vi "TreeController.vi"(8 "SaveHistory":bool, 10 "Tree Refnum":refnum<vi>, 11 "Commands":refnum<queue>) -> ()   [LabVIEW 2021, in "Tree.lvlib" / "Tree.lvclass"]
uses:
  Tree.lvclass
  TreeController.ctl
  TreeData.ctl
  <vilib>/Utility/miscctls.llb/LVNodeAndColumnTypeDef.ctl
  Tree.lvclass/Tree.ctl
panel:
  in  "exit":bool
  in  "Cluster":T1
  out "Mode":enum8{"AND", "OR", "NOT AND", "NOT OR"}(ring)
  out "Filter":cluster{"Matches String":string, "Column":i32}[](array[cluster])
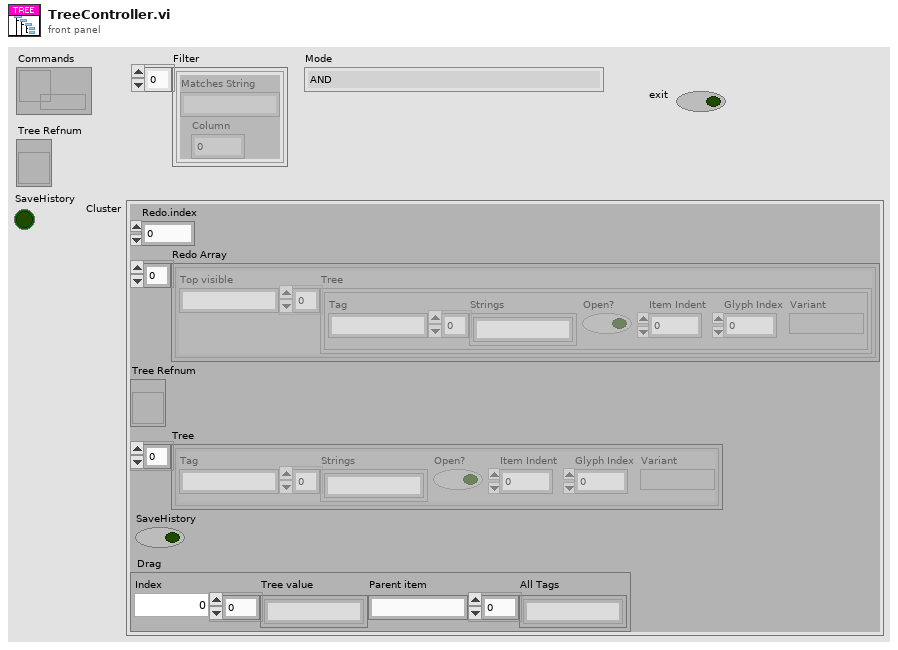
[diagram p1: front panel]
types:
  T1 = typedef "Tree.lvlib/Tree.lvclass/TreeController.ctl" = cluster{"Redo.index":i32, "Redo Array":cluster{"Top visible":string, "Tree":T2[]}[], "Tree Refnum":refnum<vi>, "Tree":T2[], "SaveHistory":bool, "Drag":cluster{"Index":i32, "Tree value":string[], "Parent item":string, "All Tags":string[]}}
  T2 = typedef "Tree.lvlib/Tree.lvclass/TreeData.ctl" = cluster{"Tag":string, "Strings":string[], "Open?":bool, "Item Indent":i32, "Glyph Index":i32, "Variant":variant}
  T3 = cluster{"NewElement":cluster{"SelectedTag":string, "New Tag":string, "Strings":string[], "Child?":bool, "Variant":variant}, "queue out":refnum<queue>}
  T4 = cluster{"Tag":string[], "queue out":refnum<queue>}
  T5 = cluster{"Tag":string, "Strings":string[], "Open?":bool, "Item Indent":i32, "Glyph Index":i32, "Variant":variant}
  T6 = cluster{"Tree":T2[], "Mode":enum16{"Clear & Insert", "Update Existing", "Add to End"}}
  T7 = cluster{"Tags":string[], "queue out":refnum<queue>}
  T8 = cluster{"cluster":cluster{enum16{"EditStrings", "EditGraph", "EditVariant"}, "Tag":string, "Value":variant}, "queue out":refnum<queue>}
  T9 = cluster{"T=Back F=Forward":bool, "queue out":refnum<queue>}
  T10 = typedef "LVNodeAndColumnTypeDef.ctl" = cluster{"Node":string, "Column":i32}
  T11 = enum8{"Enabled", "Disabled", "Disabled and Grayed Out"}
  T12 = cluster{"Mode":enum8{"AND", "OR", "NOT AND", "NOT OR"}, "Filter":cluster{"Matches String":string, "Column":i32}[], "Show Hierarhy":cluster{"Show hierarhy in first column(F)":bool, "Left separator":string, "Right separator":string}}
  T13 = cluster{"SelectedTag":string, "New Tag":string, "Strings":string[], "Child?":bool, "Variant":variant}
  T14 = cluster{"StepBack":enum8{"Enabled", "Disabled", "Disabled and Grayed Out"}, "StepForward":enum8{"Enabled", "Disabled", "Disabled and Grayed Out"}, "Edit Tree Items:Add Item":string}
  T15 = cluster{"StepBack":enum8{"Enabled", "Disabled", "Disabled and Grayed Out"}, "StepForward":enum8{"Enabled", "Disabled", "Disabled and Grayed Out"}}
  T16 = cluster{"Node":string, cluster{"Tag":string, "Strings":string[], "Open?":bool, "Item Indent":i32, "Glyph Index":i32, "Variant":variant}[]}
  T17 = enum16{"Clear & Insert", "Update Existing", "Add to End"}
  T18 = cluster{enum16{"EditStrings", "EditGraph", "EditVariant"}, "Tag":string, "Value":variant}
  T19 = enum16{"EditStrings", "EditGraph", "EditVariant"}
  T20 = cluster{"Disabled & Grayed":enum8{"Enabled", "Disabled", "Disabled and Grayed Out"}, "Disabled & Grayed":enum8{"Enabled", "Disabled", "Disabled and Grayed Out"}}
  T21 = cluster{"Show hierarhy in first column(F)":bool, "Left separator":string, "Right separator":string}
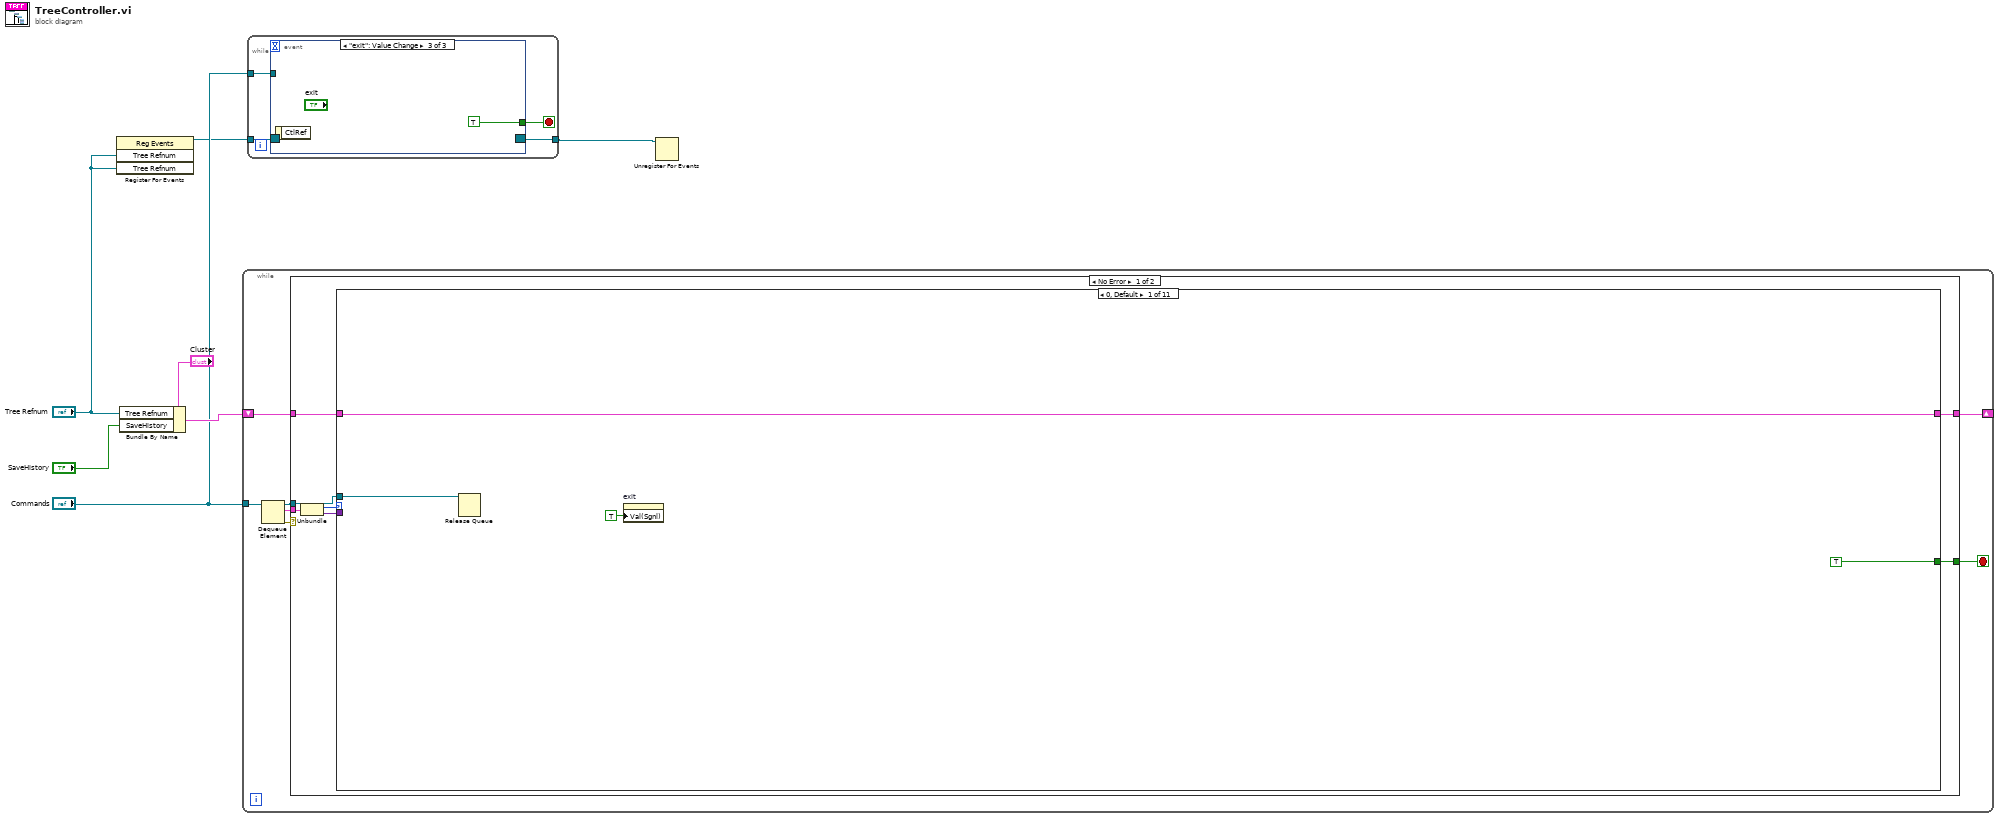
[diagram p0: block diagram]
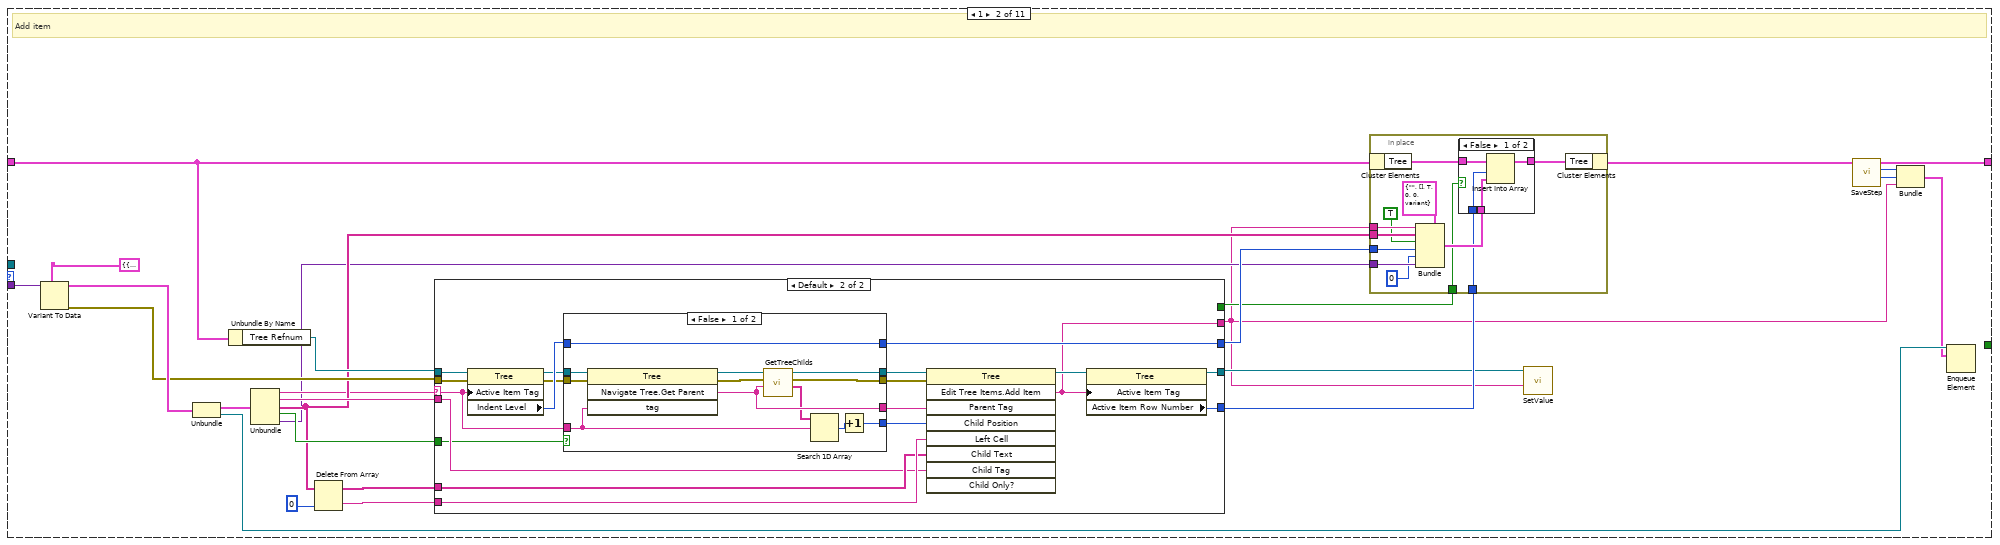
[diagram p2: hidden frame]
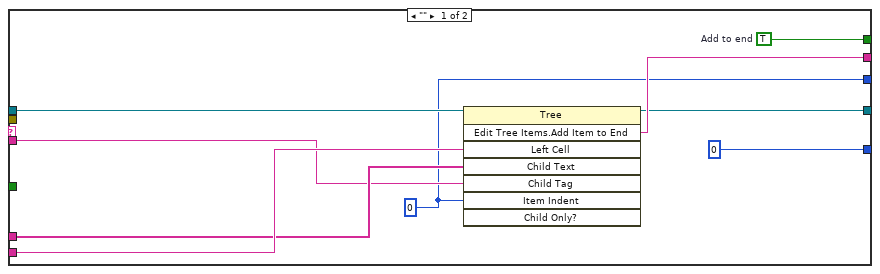
[diagram p3: hidden frame]
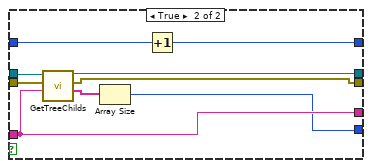
[diagram p4: hidden frame]
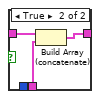
[diagram p5: hidden frame]
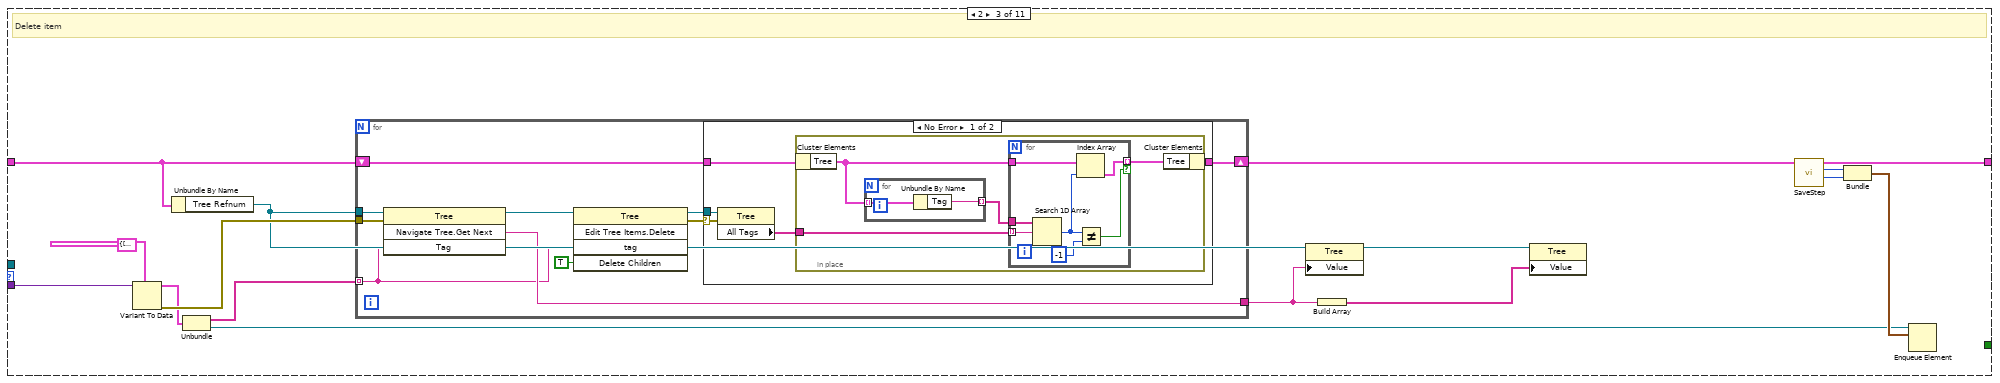
[diagram p6: hidden frame]
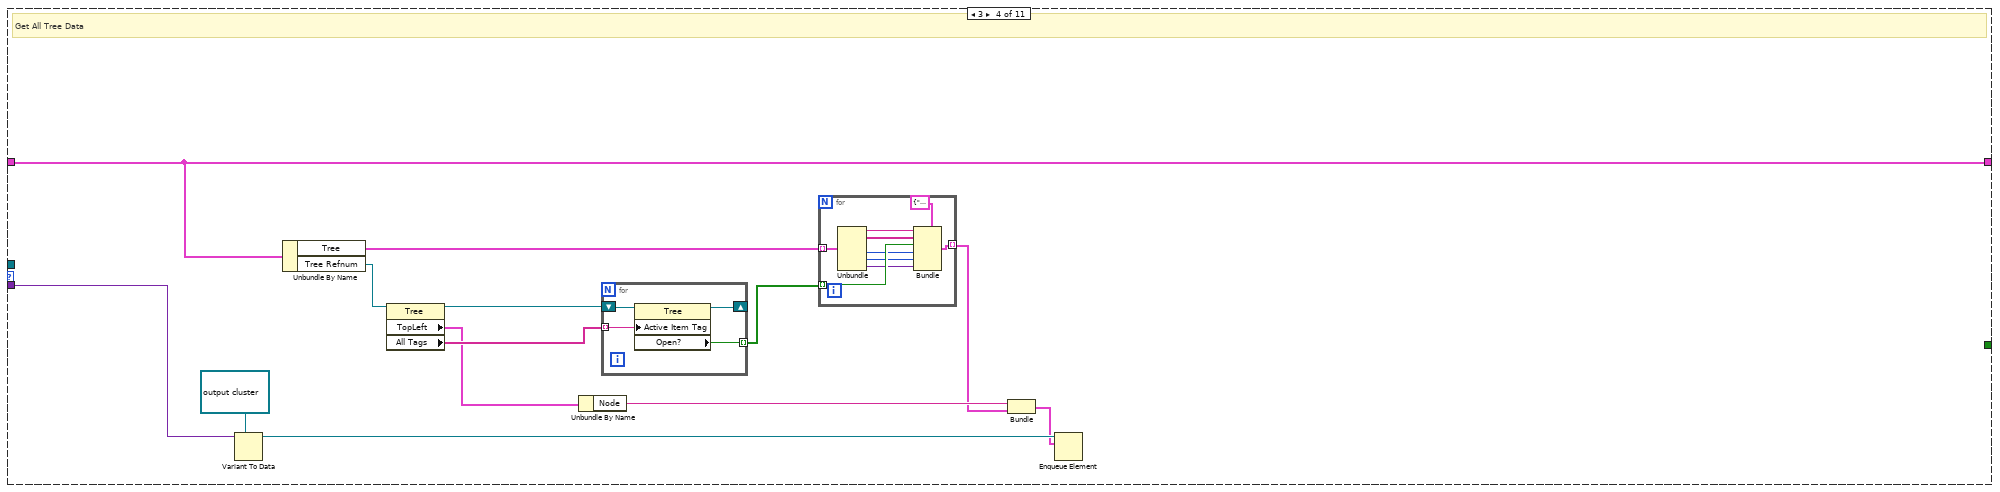
[diagram p8: hidden frame]
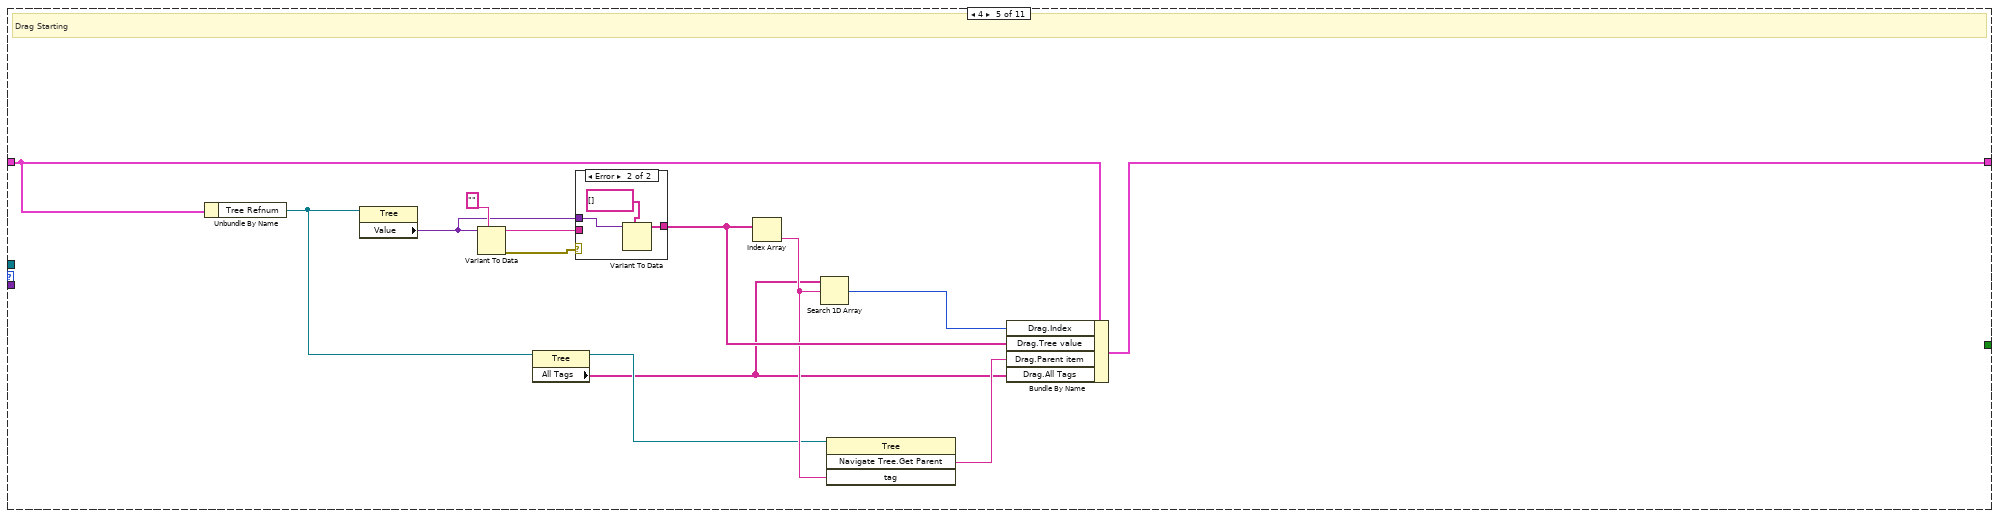
[diagram p9: hidden frame]
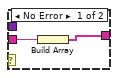
[diagram p10: hidden frame]
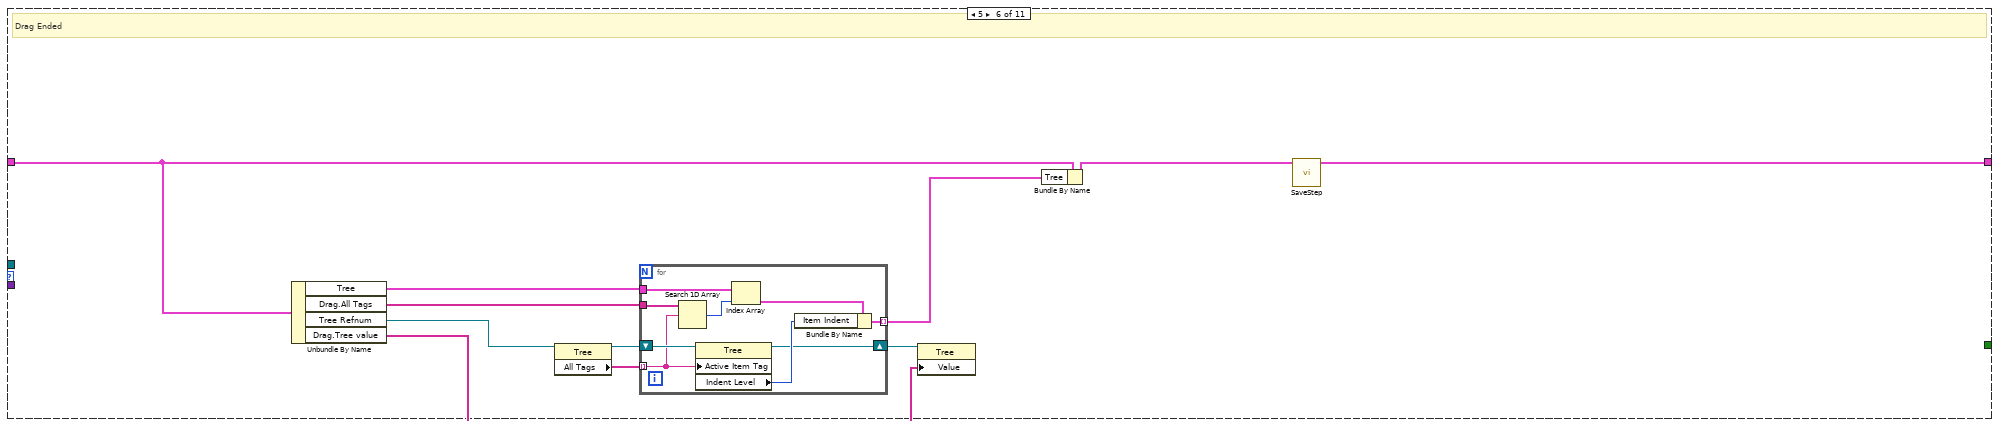
[diagram p11: hidden frame]
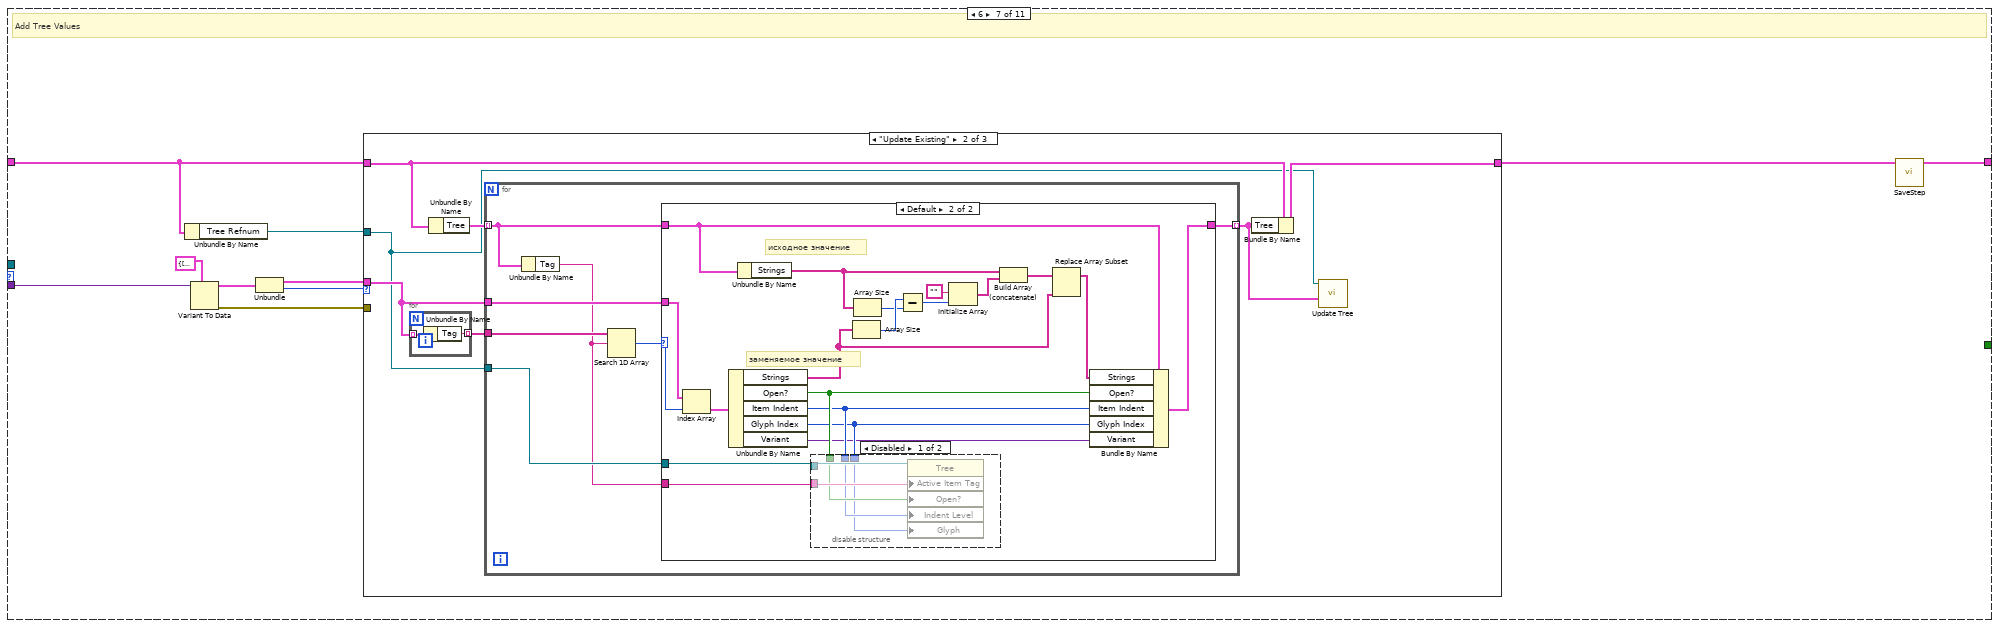
[diagram p12: hidden frame]
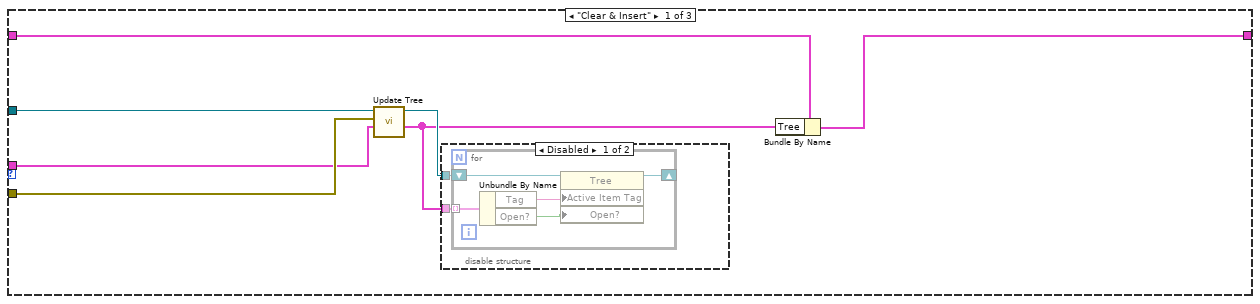
[diagram p13: hidden frame]
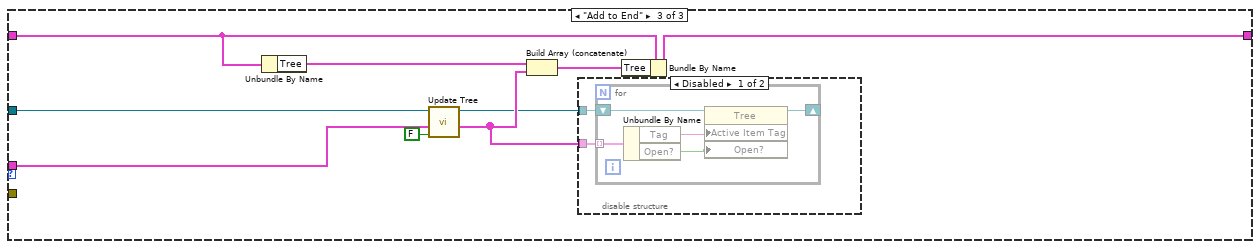
[diagram p17: hidden frame]
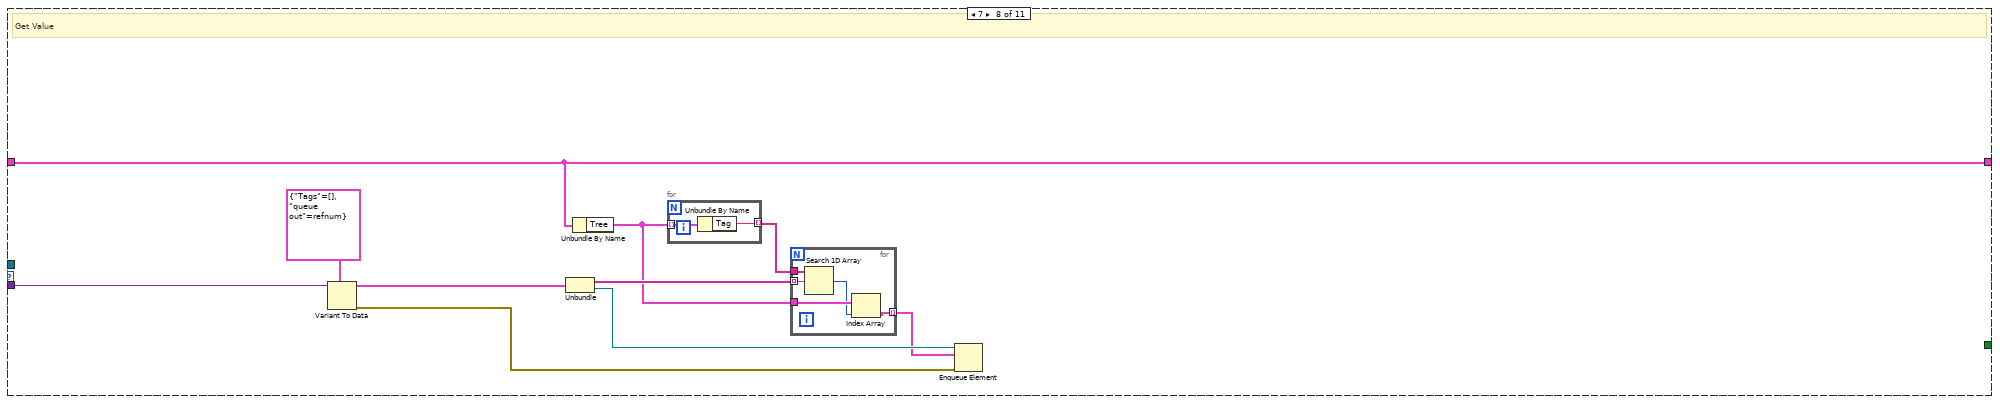
[diagram p19: hidden frame]
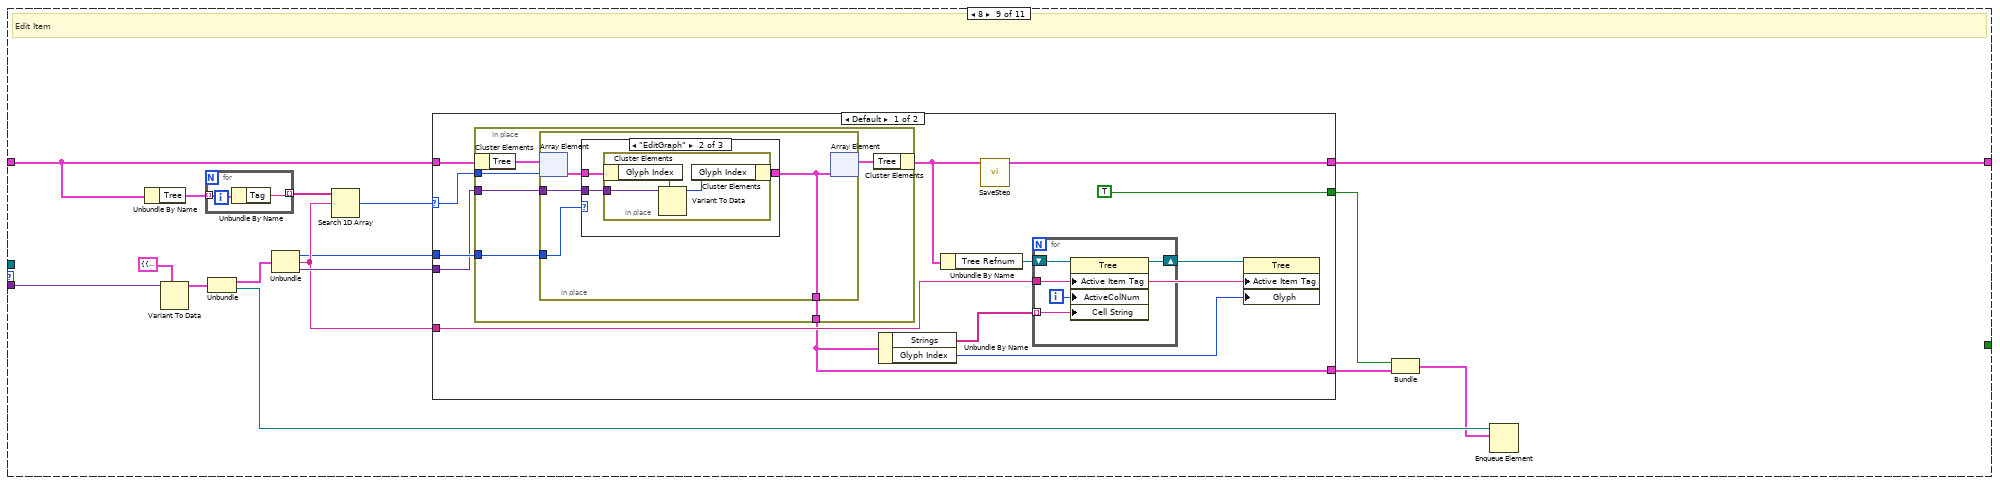
[diagram p20: hidden frame]
diagram:
  n1 = register-events("Tree Refnum", "Tree Refnum") -> (reference out=w2:refnum<event-registration>)  [unwired: 2 in, 1 out]
  n2 = Bundle By Name(cluster="Cluster", "Tree Refnum"="Tree Refnum", "SaveHistory"="SaveHistory") -> (w6:T1)
  n3 = while {
    tunnel: "Commands" -> [w14]
    shift-right: [w12] -> _
    shift-left: w6 -> [w11]
    stop <- w9 stop-if-true
    n4 = Dequeue Element(queue=w14) -> (queue out=w8:refnum<queue>, element=w13:cluster{"Tag":u8, "Value":variant}, error out=w10:errorcluster)  [unwired: 2 in, 1 out]
    n5 = case shown="No Error" w10 {
      selector: w10 -> [_ w508]
      tunnel: w13 -> [w21 _]
      tunnel: [w19 w510] -> w12
      tunnel: w11 -> [w18 w510]
      tunnel: [w16 TRUE] -> w9
      tunnel: w8 -> [w15 _]
      frame No Error {
        n6 = Unbundle(w21) -> ("Tag"=w20:u8, "Value"=w17:variant)
        n7 = case shown="0, Default" w20 {
          tunnel: [w23 w50 w132 w177 w198 w219 w235 w318 w337 w410 w449] -> w19
          tunnel: w18 -> [w23 w51 w134 w177 w203 w218 w238 w318 w338 w423 w449]
          tunnel: w17 -> [_ w49 w135 w173 _ _ w234 w320 w343 w424 w445]
          tunnel: [TRUE _ _ _ _ _ _ _ _ _ _] -> w16
          tunnel: w15 -> [w24 _ _ _ _ _ _ _ _ _ _]
          frame 0, Default {
            n8 = Release Queue(queue=w24) -> ()  [unwired: 2 in, 3 out]
            n9 = property on="exit" class="Bool (strict)"("Val(Sgnl)"=TRUE ("Value (Signaling)")) -> ()  [unwired: 2 in, 2 out]
          }
          frame 1 {
            # "Add item"
            n10 = Variant To Data(type=T3 {"NewElement"={"SelectedTag"="", "New Tag"="", "Strings"=[], "Child?"=FALSE, "Variant"=variant}, "queue out"=refnum} ("output cluster"), Variant=w49) -> (data=w48:T3, error out=w46:errorcluster)  [unwired: 1 in]
            n11 = Unbundle(w48) -> ("NewElement"=w35:T13, "queue out"=w36:refnum<queue>)
            n12 = Unbundle By Name(w51) -> ("Tree Refnum"=w38:refnum<vi>)
            n13 = Unbundle(w35) -> ("SelectedTag"=w29:string, "New Tag"=w42:string, "Strings"=w30:string[], "Child?"=w39:bool, "Variant"=w28:variant)
            n14 = Delete From Array(array=w30, index=0) -> (deleted portion=w45:string, array with subset deleted=w44:string[])  [unwired: 1 in]
            n15 = case shown="Default" w29 {
              selector: w29 -> [_ w62]
              tunnel: w45 -> [w59 w79]
              tunnel: w44 -> [w58 w78]
              tunnel: [w53 w77] -> w43
              tunnel: w42 -> [w54 w76]
              tunnel: [0 ("Active Item Row Number") w75] -> w41
              tunnel: w39 -> [_ w69]
              tunnel: w38 -> [w56 w68]
              tunnel: w46 -> [_ w64]
              tunnel: [w57 w63] -> w26
              tunnel: [w55 _] -> w34
              tunnel: [w52 w61] -> w27
              frame "" {
                w55 = TRUE  # Add to end
                w53 = 0 ("New Item Indentation")
                n16 = invoke class="Tree" method="Edit Tree Items.Add Item to End"(reference=w56, "Left Cell"=w59, "Child Text"=w58, "Child Tag"=w54, "Item Indent"=w53) -> (reference out=w52:refnum<vi>, "Edit Tree Items:Add Item to End"=w57:string)  [unwired: 3 in, 6 out]
              }
              frame Default {
                n17 = property class="Tree"(reference=w68, error in=w64, "Active Item Tag"=w62) -> (reference out=w66:refnum<vi>, error out=w65:errorcluster, "Indent Level"=w67:i32)
                n18 = case shown="False" w69 {
                  tunnel: [w80 w92] -> w77
                  tunnel: w65 -> [w89 w94]
                  tunnel: w62 -> [w91 w99]
                  tunnel: w66 -> [w90 w100]
                  tunnel: [w87 w99] -> w74
                  tunnel: [w85 w95] -> w73
                  tunnel: [w84 w96] -> w72
                  tunnel: [w81 w97] -> w71
                  tunnel: w67 -> [w80 w93]
                  frame False {
                    n19 = invoke class="Tree" method="Navigate Tree.Get Parent"(reference=w90, error in=w89, "tag"=w91) -> (reference out=w88:refnum<vi>, error out=w86:errorcluster, "Navigate Tree:Get Parent"=w87:string)  [unwired: 1 in, 1 out]
                    n20 = call "GetTreeChilds.vi"("Tag"=w87, "error in (no error)"=w86, "Tree Refnum"=w88) -> ("Childs"=w83:string[], "error out"=w85:errorcluster, "Tree Refnum"=w84:refnum<vi>)  [unwired: 6 in]
                    n21 = Search 1D Array(1D array=w83, element=w91) -> (index of element=w82:i32)  [unwired: 1 in]
                    n22 = Increment(x=w82) -> (x+1=w81:i32)
                  }
                  frame True {
                    n23 = call "GetTreeChilds.vi"("Tag"=w99, "error in (no error)"=w94, "Tree Refnum"=w100) -> ("Childs"=w98:string[], "error out"=w95:errorcluster, "Tree Refnum"=w96:refnum<vi>)  [unwired: 6 in]
                    n24 = Array Size(array=w98) -> (size(s)=w97:i32)
                    n25 = Increment(x=w93) -> (x+1=w92:i32)
                  }
                }
                n26 = invoke class="Tree" method="Edit Tree Items.Add Item"(reference=w72, error in=w73, "Parent Tag"=w74, "Child Position"=w71, "Left Cell"=w79, "Child Text"=w78, "Child Tag"=w76) -> (reference out=w70:refnum<vi>, "Edit Tree Items:Add Item"=w63:string)  [unwired: 2 in, 7 out]
                n27 = property class="Tree"(reference=w70, "Active Item Tag"=w63) -> (reference out=w61:refnum<vi>, "Active Item Row Number"=w75:i32)  [unwired: 1 in, 1 out]
              }
            }
            n28 = in-place {
              in-place-border: w26 -> [w111]
              in-place-border: w30 -> [w110]
              in-place-border: w43 -> [w109]
              in-place-border: w41 -> [w106]
              in-place-border: w34 -> [w105]
              in-place-border: w28 -> [w104]
              n29 = in-place-cluster #1(w51) -> ("Tree"=w112:T2[])
              n30 = Bundle(cluster=T2 {"Tag"="", "Strings"=[], "Open?"=TRUE, "Item Indent"=0, "Glyph Index"=0, "Variant"=variant} ("Item"), "Tag"=w111, "Strings"=w110, "Open?"=TRUE, "Item Indent"=w109, "Glyph Index"=0, "Variant"=w104) -> (w108:T2)
              n31 = case shown="False" w105 {
                tunnel: w112 -> [w116 w119]
                tunnel: w108 -> [w115 w118]
                tunnel: [w114 w117] -> w107
                tunnel: w106 -> [w113 _]
                frame False {
                  n32 = Insert Into Array(array=w116, index=w113, new element=w115) -> (w114:T2[])
                }
                frame True {
                  n33 = Build Array (concatenate)(w119, w118) -> (w117:T2[])
                }
              }
              n34 = in-place-cluster #1("Tree"=w107) -> (w37:T1)
            }
            n35 = call "SetValue.vi"("Edit Tree Items:Add Item"=w26, "TreeControl in"=w27) -> ()  [unwired: 9 in, 1 out]
            n36 = call "SaveStep.vi"("Cluster"=w37) -> ("StepForward"=w32:T11, "StepBack"=w33:T11, "Cluster"=w50:T1)  [unwired: 8 in]
            n37 = Bundle("StepBack"=w33, "StepForward"=w32, "Edit Tree Items:Add Item"=w26) -> (w31:T14)  [unwired: 1 in]
            n38 = Enqueue Element(queue=w36, element=w31) -> ()  [unwired: 2 in, 3 out]
          }
          frame 2 {
            # "Delete item"
            n39 = Variant To Data(type=T4 {"Tag"=[], "queue out"=refnum}, Variant=w135) -> (data=w130:T4, error out=w133:errorcluster)  [unwired: 1 in]
            n40 = Unbundle By Name(w134) -> ("Tree Refnum"=w121:refnum<vi>)
            n41 = Unbundle(w130) -> ("Tag"=w129:string[], "queue out"=w125:refnum<queue>)
            n42 = for {
              tunnel: w121 -> [w140]
              tunnel: w133 -> [w138]
              tunnel: w129 -> [w136] mode=indexing
              shift-right: [w142] -> w124
              shift-left: w134 -> [w144]
              tunnel: [w137] -> w122
              n43 = invoke class="Tree" method="Navigate Tree.Get Next"(reference=w140, error in=w138, "Tag"=w136) -> (reference out=w139:refnum<vi>, "Navigate Tree:Get Next Item"=w137:string)  [unwired: 1 in, 2 out]
              n44 = invoke class="Tree" method="Edit Tree Items.Delete"(reference=w139, "tag"=w136, "Delete Children"=TRUE ("Delete Children?")) -> (reference out=w143:refnum<vi>, error out=w141:errorcluster)  [unwired: 2 in, 3 out]
              n45 = case shown="No Error" w141 {
                selector: w141 -> [w146 _]
                tunnel: w144 -> [w150 w164]
                tunnel: w143 -> [w149 _]
                tunnel: [w147 w164] -> w142
                frame No Error {
                  n46 = property class="Tree"(reference=w149, error in=w146) -> ("All Tags"=w148:string[])  [unwired: 2 out]
                  n47 = in-place {
                    in-place-border: w148 -> [w154]
                    n48 = in-place-cluster #2(w150) -> ("Tree"=w152:T2[])
                    n49 = for {
                      tunnel: w152 -> [w163] mode=indexing
                      tunnel: [w162] -> w153 mode=indexing
                      n50 = Unbundle By Name(w163) -> ("Tag"=w162:string)
                    }
                    n51 = for {
                      tunnel: w154 -> [w160] mode=indexing
                      tunnel: w153 -> [w161]
                      tunnel: w152 -> [w159]
                      tunnel: [w158] -> w151 mode=indexing if=w155
                      n52 = Search 1D Array(1D array=w161, element=w160) -> (index of element=w157:i32)  [unwired: 1 in]
                      n53 = Index Array(array=w159, index=w157) -> (element=w158:T2)
                      n54 = Not Equal?(x=w157, y=-1) -> (x != y?=w155:bool)
                    }
                    n55 = in-place-cluster #2("Tree"=w151) -> (w147:T1)
                  }
                }
                frame Error {
                }
              }
            }
            n56 = property class="Tree"(reference=w121, "Value"=w122) -> (reference out=w120:refnum<vi>)  [unwired: 1 in, 1 out]
            n57 = Build Array(w122) -> (w123:string[])
            n58 = property class="Tree"(reference=w120, "Value"=w123) -> ()  [unwired: 1 in, 2 out]
            n59 = call "SaveStep.vi"("Cluster"=w124) -> ("StepForward"=w126:T11, "StepBack"=w127:T11, "Cluster"=w132:T1)  [unwired: 8 in]
            n60 = Bundle("StepBack"=w127, "StepForward"=w126) -> (w128:T15)  [unwired: 1 in]
            n61 = Enqueue Element(queue=w125, element=w128) -> ()  [unwired: 2 in, 3 out]
          }
          frame 3 {
            # "Get All Tree Data"
            n62 = Variant To Data(type=refnum<queue> refnum ("queue out"), Variant=w173) -> (data=w172:refnum<queue>)  [unwired: 1 in, 1 out]
            n63 = Unbundle By Name(w177) -> ("Tree"=w170:T2[], "Tree Refnum"=w174:refnum<vi>)
            n64 = property class="Tree"(reference=w174) -> (reference out=w175:refnum<vi>, "TopLeft"=w171:T10, "All Tags"=w176:string[])  [unwired: 1 in, 1 out]
            n65 = Unbundle By Name(w171) -> ("Node"=w168:string)
            n66 = for {
              tunnel: w176 -> [w190] mode=indexing
              shift-right: [w188] -> _
              shift-left: w175 -> [w189]
              tunnel: [w187] -> w169 mode=indexing
              n67 = property class="Tree"(reference=w189, "Active Item Tag"=w190) -> (reference out=w188:refnum<vi>, "Open?"=w187:bool)  [unwired: 1 in, 1 out]
            }
            n68 = for {
              tunnel: w170 -> [w185] mode=indexing
              tunnel: w169 -> [w184] mode=indexing
              tunnel: [w182] -> w167 mode=indexing
              n69 = Unbundle(w185) -> ("Tag"=w178:string, "Strings"=w179:string[], "Item Indent"=w183:i32, "Glyph Index"=w180:i32, "Variant"=w181:variant)  [unwired: 1 out]
              n70 = Bundle(cluster=T5 {"Tag"="", "Strings"=[], "Open?"=FALSE, "Item Indent"=0, "Glyph Index"=0, "Variant"=variant} ("Cluster"), "Tag"=w178, "Strings"=w179, "Open?"=w184, "Item Indent"=w183, "Glyph Index"=w180, "Variant"=w181) -> (w182:T5)
            }
            n71 = Bundle("Node"=w168, w167) -> (w165:T16)  [unwired: 1 in]
            n72 = Enqueue Element(queue=w172, element=w165) -> ()  [unwired: 2 in, 3 out]
          }
          frame 4 {
            # "Drag Starting"
            n73 = Unbundle By Name(w203) -> ("Tree Refnum"=w195:refnum<vi>)
            n74 = property on="Property Node" class="Tree"(reference=w195) -> ("Value"=w200:variant)  [unwired: 1 in, 2 out]
            n75 = Variant To Data(type="", Variant=w200) -> (data=w199:string, error out=w201:errorcluster)  [unwired: 1 in]
            n76 = property class="Tree"(reference=w195) -> (reference out=w192:refnum<vi>, "All Tags"=w191:string[])  [unwired: 1 in, 1 out]
            n77 = case shown="Error" w201 {
              tunnel: w200 -> [_ w208]
              tunnel: [w204 w206] -> w196
              tunnel: w199 -> [w205 _]
              frame No Error {
                n78 = Build Array(w205) -> (w204:string[])
              }
              frame Error {
                n79 = Variant To Data(type=string[] [], Variant=w208) -> (data=w206:string[])  [unwired: 1 in, 1 out]
              }
            }
            n80 = Index Array(array=w196) -> (element=w194:string)  [unwired: 1 in]
            n81 = Search 1D Array(1D array=w191, element=w194) -> (index of element=w197:i32)  [unwired: 1 in]
            n82 = invoke class="Tree" method="Navigate Tree.Get Parent"(reference=w192, "tag"=w194) -> ("Navigate Tree:Get Parent"=w193:string)  [unwired: 2 in, 3 out]
            n83 = Bundle By Name(cluster=w203, "Drag.Index"=w197, "Drag.Tree value"=w196, "Drag.Parent item"=w193, "Drag.All Tags"=w191) -> (w198:T1)
          }
          frame 5 {
            # "Drag Ended"
            n84 = Unbundle By Name(w218) -> ("Tree"=w216:T2[], "Drag.All Tags"=w215:string[], "Tree Refnum"=w217:refnum<vi>, "Drag.Tree value"=w210:string[])
            n85 = property on="Property Node" class="Tree"(reference=w217) -> (reference out=w213:refnum<vi>, "All Tags"=w214:string[])  [unwired: 1 in, 1 out]
            n86 = for {
              tunnel: w216 -> [w228]
              tunnel: w215 -> [w227]
              tunnel: w214 -> [w225] mode=indexing
              tunnel: [w221] -> w209 mode=indexing
              shift-right: [w220] -> w211
              shift-left: w213 -> [w226]
              n87 = Search 1D Array(1D array=w227, element=w225) -> (index of element=w224:i32)  [unwired: 1 in]
              n88 = property on="Property Node" class="Tree"(reference=w226, "Active Item Tag"=w225) -> (reference out=w220:refnum<vi>, "Indent Level"=w222:i32)  [unwired: 1 in, 1 out]
              n89 = Index Array(array=w228, index=w224) -> (element=w223:T2)
              n90 = Bundle By Name(cluster=w223, "Item Indent"=w222) -> (w221:T2)
            }
            n91 = property class="Tree"(reference=w211, "Value"=w210) -> ()  [unwired: 1 in, 2 out]
            n92 = Bundle By Name(cluster=w218, "Tree"=w209) -> (w212:T1)
            n93 = call "SaveStep.vi"("Cluster"=w212) -> ("Cluster"=w219:T1)  [unwired: 8 in, 2 out]
          }
          frame 6 {
            # "Add Tree Values"
            n94 = Unbundle By Name(w238) -> ("Tree Refnum"=w237:refnum<vi>)
            n95 = Variant To Data(type=T6 {"Tree"=[], "Mode"=enum."Clear & Insert"} ("output cluster"), Variant=w234) -> (data=w232:T6, error out=w230:errorcluster)  [unwired: 1 in]
            n96 = Unbundle(w232) -> ("Tree"=w231:T2[], "Mode"=w229:T17)
            n97 = case shown="\"Update Existing\"" w229 {
              tunnel: w238 -> [w245 w259 w300]
              tunnel: w237 -> [w244 w253 w301]
              tunnel: [w243 w257 w298] -> w236
              tunnel: w231 -> [w241 w255 w303]
              tunnel: w230 -> [w242 _ _]
              frame "Clear & Insert" {
                n98 = call "Update Tree.vi"("Tree"=w241, "Error"=w242, "Tree Refnum"=w244) -> ("Tree"=w239:T2[], "Tree Refnum"=w240:refnum<vi>)  [unwired: 5 in, 2 out]
                n99 = disable-structure shown="Disabled" {
                  disable-tunnel: w240 -> [w247 _]
                  disable-tunnel: w239 -> [w246 _]
                  frame Disabled {
                    n100 = for {
                      shift-right: [w251] -> _
                      shift-left: w247 -> [w252]
                      tunnel: w246 -> [w250] mode=indexing
                      n101 = Unbundle By Name(w250) -> ("Tag"=w249:string, "Open?"=w248:bool)
                      n102 = property class="Tree"(reference=w252, "Active Item Tag"=w249, "Open?"=w248) -> (reference out=w251:refnum<vi>)  [unwired: 1 in, 1 out]
                    }
                  }
                  frame Enabled {
                  }
                }
                n103 = Bundle By Name(cluster=w245, "Tree"=w239) -> (w243:T1)
              }
              frame "Update Existing" {
                n104 = for {
                  tunnel: w255 -> [w261] mode=indexing
                  tunnel: [w260] -> w256 mode=indexing
                  n105 = Unbundle By Name(w261) -> ("Tag"=w260:string)
                }
                n106 = Unbundle By Name(w259) -> ("Tree"=w258:T2[])
                n107 = for {
                  tunnel: w258 -> [w267] mode=indexing
                  tunnel: [w268] -> w254 mode=indexing
                  tunnel: w256 -> [w266]
                  tunnel: w255 -> [w265]
                  tunnel: w253 -> [w264]
                  n108 = Unbundle By Name(w267) -> ("Tag"=w263:string)
                  n109 = Search 1D Array(1D array=w266, element=w263) -> (index of element=w262:i32)  [unwired: 1 in]
                  n110 = case shown="Default" w262 {
                    selector: w262 -> [_ w280]
                    tunnel: [w269 w289] -> w268
                    tunnel: w267 -> [w269 w279]
                    tunnel: w265 -> [_ w288]
                    tunnel: w264 -> [_ w286]
                    tunnel: w263 -> [_ w285]
                    frame -1 {
                    }
                    frame Default {
                      # "заменяемое значение"
                      # "исходное значение"
                      n111 = Index Array(array=w288, index=w280) -> (element=w287:T2)
                      n112 = Unbundle By Name(w287) -> ("Strings"=w271:string[], "Open?"=w284:bool, "Item Indent"=w283:i32, "Glyph Index"=w282:i32, "Variant"=w281:variant)
                      n113 = Unbundle By Name(w279) -> ("Strings"=w272:string[])
                      n114 = disable-structure shown="Disabled" {
                        disable-tunnel: w286 -> [w294 _]
                        disable-tunnel: w285 -> [w293 _]
                        disable-tunnel: w284 -> [w292 _]
                        disable-tunnel: w283 -> [w291 _]
                        disable-tunnel: w282 -> [w290 _]
                        frame Disabled {
                          n115 = property class="Tree"(reference=w294, "Active Item Tag"=w293, "Open?"=w292, "Indent Level"=w291, "Glyph"=w290) -> ()  [unwired: 1 in, 2 out]
                        }
                        frame Enabled {
                        }
                      }
                      n116 = Array Size(array=w271) -> (size(s)=w276:i32)
                      n117 = Array Size(array=w272) -> (size(s)=w275:i32)
                      n118 = Subtract(x=w276, y=w275) -> (x-y=w277:i32)
                      n119 = Initialize Array("", w277) -> (w274:string[])
                      n120 = Build Array (concatenate)(w272, w274) -> (w278:string[])
                      n121 = Replace Array Subset(array=w278, new element=w271) -> (w270:string[])  [unwired: 1 in]
                      n122 = Bundle By Name(cluster=w279, "Strings"=w270, "Open?"=w284, "Item Indent"=w283, "Glyph Index"=w282, "Variant"=w281) -> (w289:T2)
                    }
                  }
                }
                n123 = Bundle By Name(cluster=w259, "Tree"=w254) -> (w257:T1)
                n124 = call "Update Tree.vi"("Tree"=w254, "Tree Refnum"=w253) -> ()  [unwired: 6 in, 4 out]
              }
              frame "Add to End" {
                n125 = Unbundle By Name(w300) -> ("Tree"=w299:T2[])
                n126 = call "Update Tree.vi"("Replace? (T)"=FALSE ("Replace?"), "Tree"=w303, "Tree Refnum"=w301) -> ("Tree"=w296:T2[], "Tree Refnum"=w295:refnum<vi>)  [unwired: 5 in, 2 out]
                n127 = Build Array (concatenate)(w299, w296) -> (w297:T2[])
                n128 = disable-structure shown="Disabled" {
                  disable-tunnel: w296 -> [w305 _]
                  disable-tunnel: w295 -> [w304 _]
                  frame Disabled {
                    n129 = for {
                      shift-right: [w309] -> _
                      shift-left: w304 -> [w310]
                      tunnel: w305 -> [w308] mode=indexing
                      n130 = Unbundle By Name(w308) -> ("Tag"=w307:string, "Open?"=w306:bool)
                      n131 = property class="Tree"(reference=w310, "Active Item Tag"=w307, "Open?"=w306) -> (reference out=w309:refnum<vi>)  [unwired: 1 in, 1 out]
                    }
                  }
                  frame Enabled {
                  }
                }
                n132 = Bundle By Name(cluster=w300, "Tree"=w297) -> (w298:T1)
              }
            }
            n133 = call "SaveStep.vi"("Cluster"=w236) -> ("Cluster"=w235:T1)  [unwired: 8 in, 2 out]
          }
          frame 7 {
            # "Get Value"
            n134 = Variant To Data(type=T7 {"Tags"=[], "queue out"=refnum} ("output cluster"), Variant=w320) -> (data=w319:T7, error out=w311:errorcluster)  [unwired: 1 in]
            n135 = Unbundle(w319) -> ("Tags"=w313:string[], "queue out"=w317:refnum<queue>)
            n136 = Unbundle By Name(w318) -> ("Tree"=w312:T2[])
            n137 = for {
              tunnel: w312 -> [w327] mode=indexing
              tunnel: [w326] -> w314 mode=indexing
              n138 = Unbundle By Name(w327) -> ("Tag"=w326:string)
            }
            n139 = for {
              tunnel: w314 -> [w325]
              tunnel: w313 -> [w324] mode=indexing
              tunnel: w312 -> [w323]
              tunnel: [w321] -> w315 mode=indexing
              n140 = Search 1D Array(1D array=w325, element=w324) -> (index of element=w322:i32)  [unwired: 1 in]
              n141 = Index Array(array=w323, index=w322) -> (element=w321:T2)
            }
            n142 = Enqueue Element(queue=w317, element=w315, error in (no error)=w311) -> ()  [unwired: 1 in, 3 out]
          }
          frame 8 {
            # "Edit Item"
            n143 = Unbundle By Name(w338) -> ("Tree"=w332:T2[])
            n144 = Variant To Data(type=T8 {"cluster"={enum."EditStrings", "Tag"="", "Value"=variant}, "queue out"=refnum} ("output cluster"), Variant=w343) -> (data=w342:T8)  [unwired: 1 in, 1 out]
            n145 = for {
              tunnel: w332 -> [w390] mode=indexing
              tunnel: [w389] -> w331 mode=indexing
              n146 = Unbundle By Name(w390) -> ("Tag"=w389:string)
            }
            n147 = Unbundle(w342) -> ("cluster"=w341:T18, "queue out"=w340:refnum<queue>)
            n148 = Unbundle(w341) -> (w333:T19, "Tag"=w336:string, "Value"=w339:variant)
            n149 = Search 1D Array(1D array=w331, element=w336) -> (index of element=w330:i32)  [unwired: 1 in]
            n150 = case shown="Default" w330 {
              selector: w330 -> [w354 _]
              tunnel: [TRUE _] -> w335
              tunnel: w338 -> [w355 w388]
              tunnel: [w351 w388] -> w337
              tunnel: w333 -> [w349 _]
              tunnel: w339 -> [w348 _]
              tunnel: w336 -> [w346 _]
              tunnel: [w344 _] -> w328
              frame Default {
                n151 = in-place {
                  in-place-border: w354 -> [w365]
                  in-place-border: [w364] -> w344
                  in-place-border: w349 -> [w363]
                  in-place-border: w348 -> [w362]
                  n152 = in-place-cluster #3(w355) -> ("Tree"=w367:T2[])
                  n153 = in-place {
                    in-place-border: [w370] -> w364
                    in-place-border: w363 -> [w369]
                    in-place-border: w362 -> [w368]
                    n154 = in-place-array #4(w367, w365) -> (w371:T2)
                    n155 = case shown="\"EditGraph\"" w369 {
                      tunnel: w371 -> [w374 w380 w386]
                      tunnel: [w373 w379 w385] -> w370
                      tunnel: w368 -> [w372 w378 w384]
                      frame "EditStrings", Default {
                        n156 = in-place {
                          in-place-border: w372 -> [w377]
                          n157 = in-place-cluster #5(w374) -> ("Strings"=w375:string[])
                          n158 = Variant To Data(type=w375, Variant=w377) -> (data=w376:string[])  [unwired: 1 in, 1 out]
                          n159 = in-place-cluster #5("Strings"=w376) -> (w373:T2)
                        }
                      }
                      frame "EditGraph" {
                        n160 = in-place {
                          in-place-border: w378 -> [w383]
                          n161 = in-place-cluster #6(w380) -> ("Glyph Index"=w381:i32)
                          n162 = Variant To Data(type=w381, Variant=w383) -> (data=w382:i32)  [unwired: 1 in, 1 out]
                          n163 = in-place-cluster #6("Glyph Index"=w382) -> (w379:T2)
                        }
                      }
                      frame "EditVariant" {
                        n164 = in-place {
                          in-place-border: w384 -> [w387]
                          n165 = in-place-cluster #7(w386) -> ()  [unwired: 1 out]
                          n166 = in-place-cluster #7("Variant"=w387) -> (w385:T2)
                        }
                      }
                    }
                    n167 = in-place-array #4(w370) -> (w366:T2[])  [unwired: 1 out]
                  }
                  n168 = in-place-cluster #3("Tree"=w366) -> (w352:T1)
                }
                n169 = Unbundle By Name(w344) -> ("Strings"=w350:string[], "Glyph Index"=w345:i32)
                n170 = Unbundle By Name(w352) -> ("Tree Refnum"=w353:refnum<vi>)
                n171 = call "SaveStep.vi"("Cluster"=w352) -> ("Cluster"=w351:T1)  [unwired: 8 in, 2 out]
                n172 = for {
                  tunnel: w350 -> [w359] mode=indexing
                  tunnel: w346 -> [w358]
                  shift-right: [w357] -> w347
                  shift-left: w353 -> [w361]
                  i -> [w360]
                  n173 = property class="Tree"(reference=w361, "Active Item Tag"=w358, "ActiveColNum"=w360, "Cell String"=w359) -> (reference out=w357:refnum<vi>)  [unwired: 1 in, 1 out]
                }
                n174 = property class="Tree"(reference=w347, "Active Item Tag"=w346, "Glyph"=w345) -> ()  [unwired: 1 in, 2 out]
              }
              frame -1 {
              }
            }
            n175 = Bundle(w335, "Item"=w328) -> (w334:cluster{bool, "Item":T2})  [unwired: 1 in]
            n176 = Enqueue Element(queue=w340, element=w334) -> ()  [unwired: 2 in, 3 out]
          }
          frame 9 {
            # "StepBack"
            n177 = Unbundle By Name(w423) -> ("Redo.index"=w422:i32)
            n178 = Variant To Data(type=T9 {"T=Back F=Forward"=TRUE, "queue out"=refnum} ("output cluster"), Variant=w424) -> (data=w421:T9)  [unwired: 1 in, 1 out]
            n179 = Unbundle(w421) -> ("T=Back F=Forward"=w407:bool, "queue out"=w406:refnum<queue>)
            n180 = case shown="True" w407 {
              tunnel: [w434 w436] -> w401
              tunnel: w422 -> [w435 w437]
              frame False {
                # "forward"
                n181 = Decrement(x=w435) -> (x-1=w434:i32)
              }
              frame True {
                # "back"
                n182 = Increment(x=w437) -> (x+1=w436:i32)
              }
            }
            n183 = Bundle By Name(cluster=w423, "Redo.index"=w401) -> (w417:T1)
            n184 = Unbundle By Name(w417) -> ("Tree Refnum"=w416:refnum<vi>, "Redo Array"=w392:cluster{"Top visible":string, "Tree":T2[]}[])
            n185 = Array Size(array=w392) -> (size(s)=w420:i32)
            n186 = Subtract(x=w420, y=w401) -> (x-y=w419:i32)
            n187 = Decrement(x=w419) -> (x-1=w395:i32)
            n188 = Index Array(array=w392, index=w395) -> (element=w418:cluster{"Top visible":string, "Tree":T2[]})
            n189 = Unbundle(w418) -> ("Top visible"=w411:string, "Tree"=w397:T2[])
            n190 = call "Update Tree.vi"("Replace? (T)"=TRUE ("Replace?"), "Tree"=w397, "Tree Refnum"=w416) -> ("Tree"=w396:T2[], "Error"=w412:errorcluster, "Tree Refnum"=w413:refnum<vi>)  [unwired: 5 in, 1 out]
            n191 = Bundle By Name(cluster=T10 {"Node"="", "Column"=0} ("Top Left Visible Cell"), "Node"=w411) -> (w414:T10)
            n192 = property class="Tree"(reference=w413, error in=w412, "TopLeft"=w414) -> (reference out=w409:refnum<vi>)  [unwired: 1 out]
            n193 = for {
              shift-right: [w432] -> _
              shift-left: w409 -> [w433]
              tunnel: w396 -> [w431] mode=indexing
              n194 = Unbundle By Name(w431) -> ("Tag"=w429:string, "Open?"=w430:bool)
              n195 = property class="Tree"(reference=w433, "Active Item Tag"=w429, "Open?"=w430) -> (reference out=w432:refnum<vi>)  [unwired: 1 in, 1 out]
            }
            n196 = Array Size(array=w392) -> (size(s)=w404:i32)
            n197 = Bundle By Name(cluster=w417, "Tree"=w396) -> (w410:T1)
            n198 = Subtract(x=w404, y=w401) -> (x-y=w391:i32)
            n199 = Equal To 0?(x=w404) -> (x = 0?=w393:bool)
            n200 = Equal To 0?(x=w391) -> (x = 0?=w405:bool)
            n201 = Equal To 0?(x=w401) -> (x = 0?=w402:bool)
            n202 = Or(x=w393, y=w405) -> (x .or. y?=w403:bool)
            n203 = case shown="True" w403 {
              tunnel: [T11."Enabled" ("Disabled & Grayed") T11."Disabled and Grayed Out" ("Disabled & Grayed")] -> w400
              frame False {
              }
              frame True {
              }
            }
            n204 = case shown="True" w402 {
              tunnel: [T11."Enabled" ("Disabled & Grayed") T11."Disabled and Grayed Out" ("Disabled & Grayed")] -> w399
              frame False {
              }
              frame True {
              }
            }
            n205 = Bundle("Disabled & Grayed"=w400, "Disabled & Grayed"=w399) -> (w398:T20)  [unwired: 1 in]
            n206 = Enqueue Element(queue=w406, element=w398) -> ()  [unwired: 2 in, 3 out]
          }
          frame 10 {
            # "Filter"
            n207 = Variant To Data(type=T12 {"Mode"=enum."AND", "Filter"=[], "Show Hierarhy"={"Show hierarhy in first column(F)"=FALSE, "Left separator"="", "Right separator"=""}} ("output cluster"), Variant=w445) -> (data=w444:T12)  [unwired: 1 in, 1 out]
            n208 = Unbundle(w444) -> ("Mode"=w440:enum8{"AND", "OR", "NOT AND", "NOT OR"}, "Filter"=w439:cluster{"Matches String":string, "Column":i32}[], "Show Hierarhy"=w441:T21)
            "Filter" <- w439
            "Mode" <- w440
            n209 = Empty Array?(array=w439) -> (empty?=w438:bool)
            n210 = Unbundle By Name(w449) -> ("Tree"=w442:T2[])
            n211 = case shown="True" w438 {
              tunnel: [w459 w507] -> w447
              tunnel: w442 -> [w454 w507]
              tunnel: w441 -> [w453 _]
              tunnel: w440 -> [w451 _]
              tunnel: w439 -> [w450 _]
              frame False {
                n212 = for {
                  tunnel: w454 -> [w461] mode=indexing
                  tunnel: [w460] -> w458 mode=indexing
                  n213 = Unbundle By Name(w461) -> ("Tag"=w460:string)
                }
                n214 = Unbundle(w453) -> ("Show hierarhy in first column(F)"=w457:bool, "Left separator"=w456:string, "Right separator"=w455:string)
                n215 = call "ApplyFilter.vi"("Filter"=w450, "Mode"=w451, "Tree"=w454) -> ("Array"=w452:T2[])  [unwired: 8 in]
                n216 = case shown="True" w457 {
                  tunnel: w452 -> [w462 w468]
                  tunnel: w454 -> [_ w467]
                  tunnel: w458 -> [_ w466]
                  tunnel: [w462 w465] -> w459
                  tunnel: w456 -> [_ w464]
                  tunnel: w455 -> [_ w463]
                  frame False {
                  }
                  frame True {
                    # "Show hierarhy in first column"
                    n217 = for {
                      tunnel: w468 -> [w483] mode=indexing
                      tunnel: w467 -> [w480]
                      tunnel: w466 -> [w485]
                      tunnel: [w482] -> w465 mode=indexing
                      tunnel: w464 -> [w472]
                      tunnel: w463 -> [w471]
                      n218 = Unbundle By Name(w483) -> ("Tag"=w484:string)
                      n219 = Search 1D Array(1D array=w485, element=w484) -> (index of element=w481:i32)  [unwired: 1 in]
                      n220 = Index Array(array=w480, index=w481) -> (element=w479:T2)
                      n221 = Unbundle By Name(w479) -> ("Strings"=w478:string[], "Item Indent"=w470:i32)
                      n222 = while {
                        tunnel: w480 -> [w496]
                        shift-right: [w488] -> _
                        shift-left: w481 -> [w497]
                        tunnel: [w491] -> w474 mode=indexing
                        tunnel: w472 -> [w490]
                        tunnel: w471 -> [w489]
                        shift-right: [w486] -> _
                        shift-left: w470 -> [w487]
                        stop <- w493 stop-if-true
                        n223 = while {
                          tunnel: w496 -> [w506]
                          tunnel: w487 -> [w503]
                          shift-right: [w500] -> w488
                          shift-left: w497 -> [w505]
                          tunnel: [w499] -> w493
                          tunnel: [w498] -> _
                          stop <- w501 stop-if-true
                          n224 = Decrement(x=w505) -> (x-1=w500:i32)
                          n225 = Index Array(array=w506, index=w500) -> (element=w504:T2)
                          n226 = Unbundle By Name(w504) -> ("Item Indent"=w498:i32)
                          n227 = Less?(x=w498, y=w503) -> (x < y?=w502:bool)
                          n228 = Equal To 0?(x=w498) -> (x = 0?=w499:bool)
                          n229 = Or(x=w499, y=w502) -> (x .or. y?=w501:bool)
                        }
                        n230 = Index Array(array=w496, index=w488) -> (element=w495:T2)
                        n231 = Decrement(x=w487) -> (x-1=w486:i32)
                        n232 = Unbundle By Name(w495) -> ("Strings"=w494:string[])
                        n233 = Index Array(array=w494) -> (element=w492:string)  [unwired: 1 in]
                        n234 = Concatenate Strings(w490, w492, w489) -> (w491:string)
                      }
                      n235 = Index Array(array=w478) -> (element=w475:string)  [unwired: 1 in]
                      n236 = Reverse 1D Array(array=w474) -> (reversed array=w469:string[])
                      n237 = Concatenate Strings(w469, w475) -> (w473:string)
                      n238 = Replace Array Subset(array=w478, new element=w473, index=0) -> (w477:string[])
                      n239 = Bundle By Name(cluster=w483, "Strings"=w477) -> (w482:T2)
                    }
                  }
                }
              }
              frame True {
                # "Отмена текущего фильра"
              }
            }
            n240 = Unbundle By Name(w449) -> ("Tree Refnum"=w446:refnum<vi>)
            n241 = call "Update Tree.vi"("Replace? (T)"=TRUE ("Replace?"), "Tree"=w447, "Tree Refnum"=w446) -> ()  [unwired: 5 in, 4 out]
          }
        }
      }
      frame Error {
        n242 = call <vilib>:"Simple Error Handler.vi"("error in (no error)"=w508) -> ()  [unwired: 4 in, 5 out]
      }
    }
  }
  n243 = while {
    tunnel: w2 -> [w514]
    tunnel: "Commands" -> [w511]
    tunnel: [w512] -> w1
    stop <- w513 stop-if-true
    n244 = event shown="[2] \"exit\": Value Change" {
      selector: w514 -> [_ _ _]
      dyn-events: [_ _ _] -> w512
      timeout: _ -> [_ _ _]
      tunnel: [_ _ TRUE] -> w513
      tunnel: w511 -> [w515 w518 _]
      event Drag Ended {
        n245 = event-data() -> ()  [unwired: 1 in, 1 out]
        n246 = Enqueue Element(queue=w515, element=cluster{"Tag":u8, "Value":variant} {"Tag"=5, "Value"=variant}) -> ()  [unwired: 2 in, 3 out]
      }
      event Drag Starting {
        n247 = event-data() -> ()  [unwired: 1 in, 1 out]
        n248 = Enqueue Element(queue=w518, element=cluster{"Tag":u8, "Value":variant} {"Tag"=4, "Value"=variant}) -> ()  [unwired: 2 in, 3 out]
      }
      event "exit": Value Change {
        n249 = event-data() -> ()  [unwired: 1 in, 1 out]
      }
    }
  }
  n250 = Unregister For Events(event registration refnum=w1) -> ()  [unwired: 1 in, 1 out]
